vi "Register1.vi"(2 "MOD":i32, 3 "Phase":i16=1) -> (0 "HEX1":u32 format="%08x", 1 "Reg 1":bool[](array[boolean]))   [LabVIEW 2017]
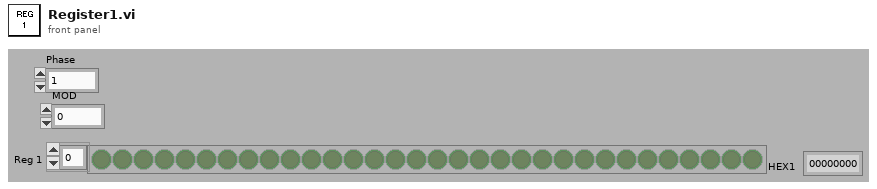
[diagram p1: front panel]
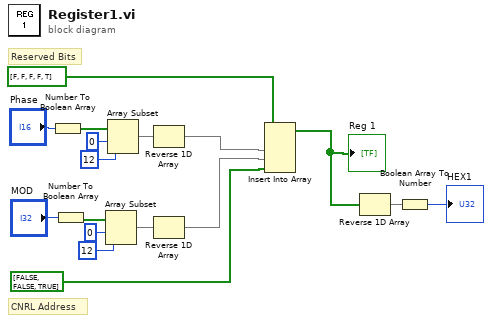
[diagram p0: block diagram]
diagram:
  # "Reserved Bits"
  # "CNRL Address"
  n1 = Number To Boolean Array(number="Phase") -> (Boolean array=w6:bool[])
  n2 = Number To Boolean Array(number="MOD") -> (Boolean array=w15:bool[])
  n3 = Array Subset(array=w15, index=0, length=12) -> (w14:bool[])
  n4 = Array Subset(array=w6, index=0, length=12) -> (w5:bool[])
  n5 = Reverse 1D Array(array=w5) -> (reversed array=w4:bool[])
  n6 = Reverse 1D Array(array=w14) -> (reversed array=w3:bool[])
  n7 = Insert Into Array(array=bool[] [FALSE, FALSE, FALSE, FALSE, TRUE], new element #1=w4, new element #2=w3, new element #3=bool[] [FALSE, FALSE, TRUE]) -> (w1:bool[])  [unwired: 1 in]
  "Reg 1" <- w1
  n8 = Reverse 1D Array(array=w1) -> (reversed array=w11:bool[])
  n9 = Boolean Array To Number(Boolean array=w11) -> (number=→"HEX1":u32)
